vi "Send BMS Telemetry.vi"   [LabVIEW 2014]
uses:
  Global Data.vi
types:
  T1 = typedef "BMS Telemetry.ctl" = cluster{"Ignition":bool, "Charger Mains":bool, "Fast Charge":bool, "Simple Charger Enabled":bool, "Car State":enum16{"Off", "On, Not Charging", "Charging", "Charging Finished", "Charging Error"}, "Charging State":enum16{"Disconnected", "Pre-charging", "Main Charging", "Balancing", "Charging Finished OK", "Charging Error"}, "Charging Stage Duration":u16, "Last Charging Error":enum16{"No Error", "Cell Voltage Too Low", "No Comm from Cells so can't start", "Maximum charging stage duration expired", "No Comm from Cels so can't balande", "Cannot set balancing voltage", "Cell temps too high", "No Comms so can't determine temp", "# of Cells Mismatch", "Cells Overvoltage", "Cell Protection Event occured."}, "Number of Detected Cells":u8, "Under-Voltage":bool, "Over-Voltage":bool, "Overheat":bool, "Leakage":bool, "No Cell Comms":bool, "Low Voltage":bool, "High Temperature":bool, "Min Cell V":dbl, "Max Cell V":dbl, "Mean Cell V":dbl, "Total V":dbl, "Min Cell t":dbl, "Max Cell t":dbl, "Mean Cell t":dbl, "Cell Voltages":cluster{"[0]":dbl, "[1]":dbl, "[2]":dbl, "[3]":dbl, "[4]":dbl, "[5]":dbl, "[6]":dbl, "[7]":dbl, "[8]":dbl, "[9]":dbl, "[10]":dbl, "[11]":dbl, "[12]":dbl, "[13]":dbl, "[14]":dbl, "[15]":dbl, "[16]":dbl, "[17]":dbl, "[18]":dbl, "[19]":dbl, "[20]":dbl, "[21]":dbl, "[22]":dbl, "[23]":dbl, "[24]":dbl, "[25]":dbl, "[26]":dbl, "[27]":dbl, "[28]":dbl, "[29]":dbl, "[30]":dbl, "[31]":dbl, "[32]":dbl, "[33]":dbl, "[34]":dbl, "[35]":dbl, "[36]":dbl, "[37]":dbl, "[38]":dbl, "[39]":dbl, "[40]":dbl, "[41]":dbl, "[42]":dbl, "[43]":dbl, "[44]":dbl, "[45]":dbl, "[46]":dbl, "[47]":dbl, "[48]":dbl, "[49]":dbl, "[50]":dbl, "[51]":dbl, "[52]":dbl, "[53]":dbl, "[54]":dbl, "[55]":dbl, "[56]":dbl, "[57]":dbl, "[58]":dbl, "[59]":dbl, "[60]":dbl, "[61]":dbl, "[62]":dbl, "[63]":dbl, "[64]":dbl, "[65]":dbl, "[66]":dbl, "[67]":dbl, "[68]":dbl, "[69]":dbl, "[70]":dbl}, "Cell Temps":cluster{"[0]":dbl, "[1]":dbl, "[2]":dbl, "[3]":dbl, "[4]":dbl, "[5]":dbl, "[6]":dbl, "[7]":dbl, "[8]":dbl, "[9]":dbl, "[10]":dbl, "[11]":dbl, "[12]":dbl, "[13]":dbl, "[14]":dbl, "[15]":dbl, "[16]":dbl, "[17]":dbl, "[18]":dbl, "[19]":dbl, "[20]":dbl, "[21]":dbl, "[22]":dbl, "[23]":dbl, "[24]":dbl, "[25]":dbl, "[26]":dbl, "[27]":dbl, "[28]":dbl, "[29]":dbl, "[30]":dbl, "[31]":dbl, "[32]":dbl, "[33]":dbl, "[34]":dbl, "[35]":dbl, "[36]":dbl, "[37]":dbl, "[38]":dbl, "[39]":dbl, "[40]":dbl, "[41]":dbl, "[42]":dbl, "[43]":dbl, "[44]":dbl, "[45]":dbl, "[46]":dbl, "[47]":dbl, "[48]":dbl, "[49]":dbl, "[50]":dbl, "[51]":dbl, "[52]":dbl, "[53]":dbl, "[54]":dbl, "[55]":dbl, "[56]":dbl, "[57]":dbl, "[58]":dbl, "[59]":dbl, "[60]":dbl, "[61]":dbl, "[62]":dbl, "[63]":dbl, "[64]":dbl, "[65]":dbl, "[66]":dbl, "[67]":dbl, "[68]":dbl, "[69]":dbl, "[70]":dbl}}
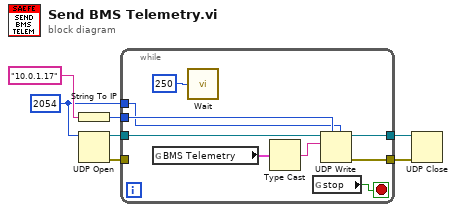
[diagram p0: block diagram]
diagram:
  w2 = u16 2054 ("port")
  n1 = String To IP(1:"10.0.1.17" ("name")) -> (0:w1:u32)
  n2 = UDP Open(11:w2) -> (port=w6:refnum<k16>, 0:w5:errorcluster)  [unwired: 4 in, 1 out]
  n3 = while {
    tunnel: w6 -> [w14]
    tunnel: w5 -> [_]
    tunnel: [w12] -> w4
    tunnel: [w11] -> w3
    tunnel: w1 -> [w10]
    tunnel: w2 -> [w9]
    stop <- w15 stop-if-true
    n4 = global read "Global Data.vi" "BMS Telemetry"() -> (w8:T1)
    n5 = call "Wait"("Count(mSec)"=u32 250) -> ()  [unwired: 1 out]
    n6 = Type Cast(x=w8) -> (*(type *) &x=w13:string)  [unwired: 1 in]
    n7 = global read "Global Data.vi" "stop"() -> (w15:bool)
    n8 = UDP Write(address=w10, port or service name=w9, connection ID=w14, data in=w13) -> (error out=w11:errorcluster, 3:w12:refnum<k16>)  [unwired: 2 in]
  }
  n9 = UDP Close(connection ID=w4, 8:w3) -> ()  [unwired: 2 out]
